vi "SIM ChkTimesteps.vi"(4 "Clock Rate (Hz)":u32, 5 "Calculate using Time Step":bool, 6 "Max TimeStep":dbl, 7 "Min TimeStep":dbl, 8 "Error In":errorcluster, 9 "Automatic Discrete Step Size?":bool, 10 "Discrete timeStep":dbl, 11 "Initial TimeStep":dbl) -> (0 "Error Out":errorcluster)   [LabVIEW 2020]
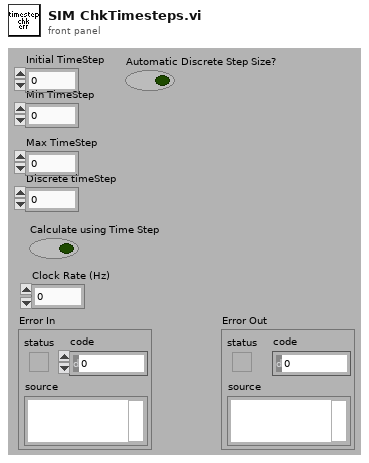
[diagram p1: front panel]
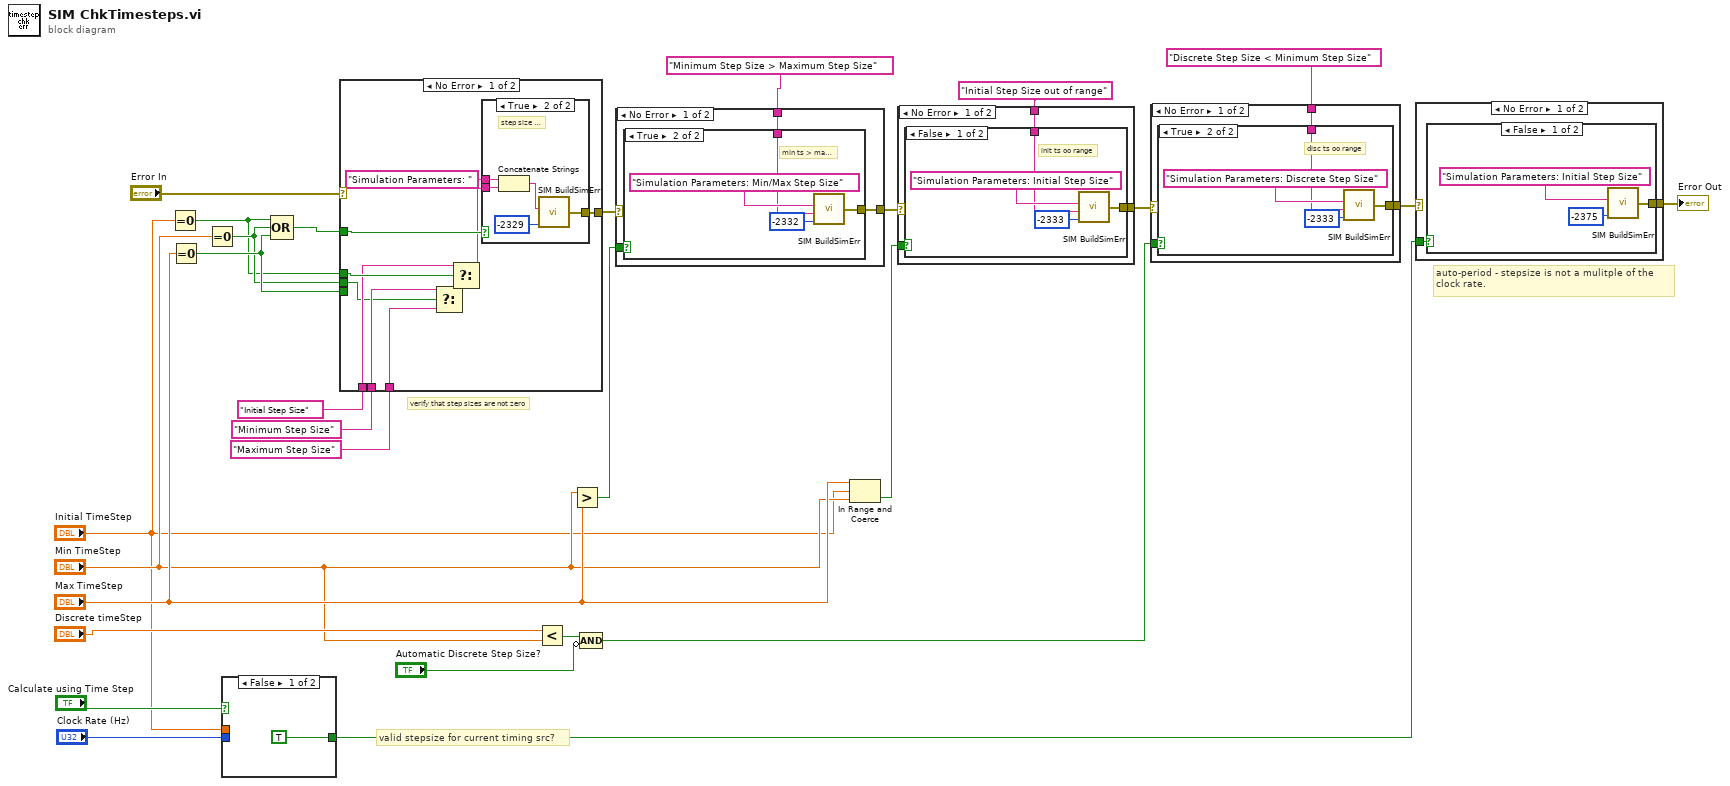
[diagram p0: block diagram]
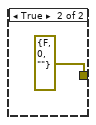
[diagram p2: hidden frame]
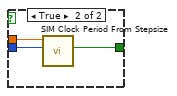
[diagram p4: hidden frame]
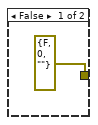
[diagram p5: hidden frame]
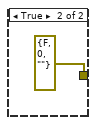
[diagram p7: hidden frame]
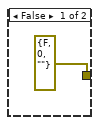
[diagram p9: hidden frame]
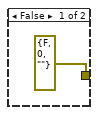
[diagram p11: hidden frame]
diagram:
  # "auto-period - stepsize is not a mulitple of the\nclock rate."
  # "valid stepsize for current timing src?"
  # "verify that step sizes are not zero"
  n1 = Equal To 0?(x="Initial TimeStep") -> (x = 0?=w26:bool)
  n2 = Equal To 0?(x="Max TimeStep") -> (x = 0?=w28:bool)
  n3 = Equal To 0?(x="Min TimeStep") -> (x = 0?=w27:bool)
  n4 = case shown="False" "Calculate using Time Step" {
    tunnel: "Clock Rate (Hz)" -> [_ w30]
    tunnel: "Initial TimeStep" -> [_ w32]
    tunnel: [TRUE ("Valid?") w31] -> w1
    frame False {
    }
    frame True {
      n5 = call "SIM Clock Period From Stepsize.vi"("Clock Rate (Hz)"=w30, "Step Size"=w32) -> ("Valid?"=w31:bool)  [unwired: 8 in, 1 out]
    }
  }
  n6 = Compound Arithmetic op=OR(w26, w27, w28) -> (w25:bool)
  n7 = case shown="No Error" "Error In" {
    selector: "Error In" -> [_ w49]
    tunnel: [w42 w49] -> w14
    tunnel: w25 -> [w41 _]
    tunnel: w26 -> [w40 _]
    tunnel: w27 -> [w37 _]
    tunnel: w28 -> [_ _]
    tunnel: "Initial Step Size" ("CallChain") -> [w39 _]
    tunnel: "Minimum Step Size" ("CallChain") -> [w38 _]
    tunnel: "Maximum Step Size" ("CallChain") -> [w33 _]
    frame No Error {
      n8 = Select(t=w38, s=w37, f=w33) -> (s? t:f=w36:string)
      n9 = Select(t=w39, s=w40, f=w36) -> (s? t:f=w35:string)
      n10 = case shown="True" w41 {
        tunnel: [errorcluster {"status"=FALSE, "code"=0, "source"=""} ("Error Cluster") w48] -> w42
        tunnel: w35 -> [_ w45]
        tunnel: "Simulation Parameters: " ("CallChain") -> [_ w46]
        frame False {
        }
        frame True {
          # "step size = 0"
          n11 = Concatenate Strings(w46, w45) -> (w44:string)
          n12 = call "SIM BuildSimErr.vi"("error.code"=-2329, "Block Name"=w44) -> ("Error Cluster"=w48:errorcluster)  [unwired: 2 in]
        }
      }
    }
    frame Error {
    }
  }
  n13 = Less?(x="Discrete timeStep", y="Min TimeStep") -> (x < y?=w8:bool)
  n14 = Greater?(x="Min TimeStep", y="Max TimeStep") -> (0:w15:bool)
  n15 = Compound Arithmetic op=AND(w8, invert "Automatic Discrete Step Size?") -> (w7:bool)
  n16 = case shown="No Error" w14 {
    selector: w14 -> [_ w58]
    tunnel: [w52 w58] -> w20
    tunnel: w15 -> [w51 _]
    tunnel: "Minimum Step Size > Maximum Step Size" ("Additional Details") -> [w50 _]
    frame No Error {
      n17 = case shown="True" w51 {
        tunnel: [errorcluster {"status"=FALSE, "code"=0, "source"=""} ("Error Cluster") w56] -> w52
        tunnel: w50 -> [_ w54]
        frame False {
        }
        frame True {
          # "min ts > max ts"
          n18 = call "SIM BuildSimErr.vi"("error.code"=-2332, "Additional Details"=w54, "Block Name"="Simulation Parameters: Min/Max Step Size" ("CallChain")) -> ("Error Cluster"=w56:errorcluster)  [unwired: 1 in]
        }
      }
    }
    frame Error {
    }
  }
  n19 = In Range and Coerce(upper limit="Max TimeStep", x="Initial TimeStep", lower limit="Min TimeStep") -> (In Range?=w13:bool)  [unwired: 1 out]
  n20 = case shown="No Error" w20 {
    selector: w20 -> [_ w67]
    tunnel: [w61 w67] -> w19
    tunnel: w13 -> [w60 _]
    tunnel: "Initial Step Size out of range" ("Additional Details") -> [w59 _]
    frame No Error {
      n21 = case shown="False" w60 {
        tunnel: [w64 errorcluster {"status"=FALSE, "code"=0, "source"=""} ("Error Cluster")] -> w61
        tunnel: w59 -> [w62 _]
        frame False {
          # "init ts oo range"
          n22 = call "SIM BuildSimErr.vi"("error.code"=-2333, "Additional Details"=w62, "Block Name"="Simulation Parameters: Initial Step Size" ("CallChain")) -> ("Error Cluster"=w64:errorcluster)  [unwired: 1 in]
        }
        frame True {
        }
      }
    }
    frame Error {
    }
  }
  n23 = case shown="No Error" w19 {
    selector: w19 -> [_ w76]
    tunnel: [w70 w76] -> w3
    tunnel: "Discrete Step Size < Minimum Step Size" ("Additional Details") -> [w69 _]
    tunnel: w7 -> [w68 _]
    frame No Error {
      n24 = case shown="True" w68 {
        tunnel: [errorcluster {"status"=FALSE, "code"=0, "source"=""} ("Error Cluster") w74] -> w70
        tunnel: w69 -> [_ w72]
        frame False {
        }
        frame True {
          # "disc ts oo range"
          n25 = call "SIM BuildSimErr.vi"("error.code"=-2333, "Additional Details"=w72, "Block Name"="Simulation Parameters: Discrete Step Size" ("CallChain")) -> ("Error Cluster"=w74:errorcluster)  [unwired: 1 in]
        }
      }
    }
    frame Error {
    }
  }
  n26 = case shown="No Error" w3 {
    selector: w3 -> [_ w83]
    tunnel: [w78 w83] -> w2
    tunnel: w1 -> [w77 _]
    frame No Error {
      n27 = case shown="False" w77 {
        tunnel: [w80 errorcluster {"status"=FALSE, "code"=0, "source"=""} ("Error Cluster")] -> w78
        frame False {
          n28 = call "SIM BuildSimErr.vi"("error.code"=-2375, "Block Name"="Simulation Parameters: Initial Step Size" ("CallChain")) -> ("Error Cluster"=w80:errorcluster)  [unwired: 2 in]
        }
        frame True {
        }
      }
    }
    frame Error {
    }
  }
  "Error Out" <- w2
